vi "GetAnglesOnSameOrder.vi"(2 "Angle 2":dbl, 3 "Angle 1":dbl) -> (0 "Wrapped A2":dbl, 1 "Wrapped A1":dbl)   [LabVIEW 2013]
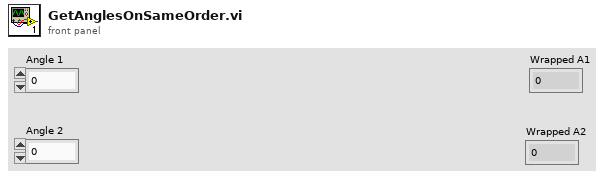
[diagram p1: front panel]
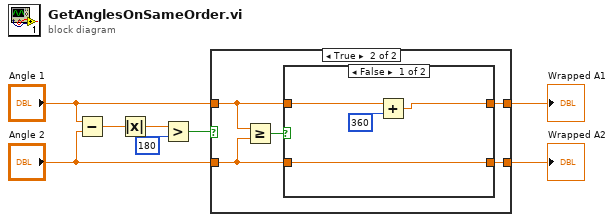
[diagram p0: block diagram]
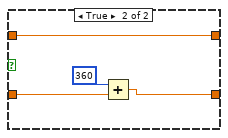
[diagram p3: hidden frame]
diagram:
  n1 = Subtract(x="Angle 1", y="Angle 2") -> (x-y=w4:dbl)
  n2 = Absolute Value(x=w4) -> (abs(x)=w6:dbl)
  n3 = Greater?(x=w6, y=180) -> (0:w1:bool)
  n4 = case shown="True" w1 {
    tunnel: "Angle 1" -> [w10 w14]
    tunnel: [w10 w13] -> w8
    tunnel: "Angle 2" -> [w9 w12]
    tunnel: [w9 w11] -> w7
    frame False {
    }
    frame True {
      n5 = Greater Or Equal?(x=w14, y=w12) -> (x >= y?=w15:bool)
      n6 = case shown="False" w15 {
        tunnel: [w17 w23] -> w13
        tunnel: w14 -> [w18 w23]
        tunnel: w12 -> [w16 w20]
        tunnel: [w16 w22] -> w11
        frame False {
          n7 = Add(x=w18, y=360) -> (x+y=w17:dbl)
        }
        frame True {
          n8 = Add(x=360, y=w20) -> (x+y=w22:dbl)
        }
      }
    }
  }
  "Wrapped A1" <- w8
  "Wrapped A2" <- w7
